vi "clone.vi"(0 "reference":refnum<class "PackageNode.lvclass">, 5 "error in (no error)":errorcluster) -> (14 "reference out":refnum<class "PackageNode.lvclass">, 15 "clonedPackageNode":refnum<class "AbstractNode.lvclass">, 19 "error out":errorcluster)   [LabVIEW 2020, in "PackageNode.lvclass"]
doc: "public Object clone()"
uses:
  <resource>/Framework/Providers/Open_GDS/UML/PackageNode_class/PackageNode.lvclass
  C:/Program Files (x86)/National Instruments/LabVIEW 2020/resource/Framework/Providers/Open_GDS/UML/RectangularNode_class/RectangularNode.lvclass
  C:/Program Files (x86)/National Instruments/LabVIEW 2020/resource/Framework/Providers/Open_GDS/UML/AbstractNode_class/AbstractNode.lvclass
  <resource>/Framework/Providers/Open_GDS/UML/AbstractNode_class/AbstractNode.lvclass
  <resource>/Framework/Providers/Open_GDS/UML/MultiLineString_class/MultiLineString.lvclass
  <resource>/Framework/Providers/Open_GDS/UML/RectangularNode_class/RectangularNode.lvclass
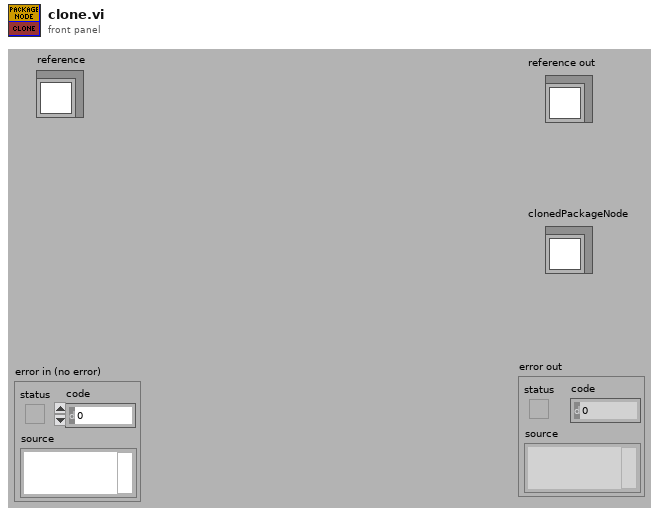
[diagram p1: front panel]
types:
  T1 = typedef "PackageNode.lvclass/ObjectAttributes.ctl" = cluster{"name":string, "contents":refnum<class "MultiLineString.lvclass">, "DEFAULT_TOP_WIDTH":i32, "DEFAULT_TOP_HEIGHT":i32, "DEFAULT_WIDTH":i32, "DEFAULT_HEIGHT":i32, "NAME_GAP":i32, "XGAP":i32, "YGAP":i32, "Collapsed":bool, "Note color":u32, "Justification":u16}
  T2 = typedef "RectangularNode.lvclass/ObjectAttributes.ctl" = cluster{"bounds":T3}
  T3 = typedef "Rectangle Rectangle2D.ctl" = cluster{"x":dbl, "y":dbl, "width":dbl, "height":dbl}
  T4 = typedef "AbstractNode.lvclass/ObjectAttributes.ctl" = cluster{"parent":refnum<class "AbstractNode.lvclass">, "children":refnum<class "AbstractNode.lvclass">[], "Hidden":bool}
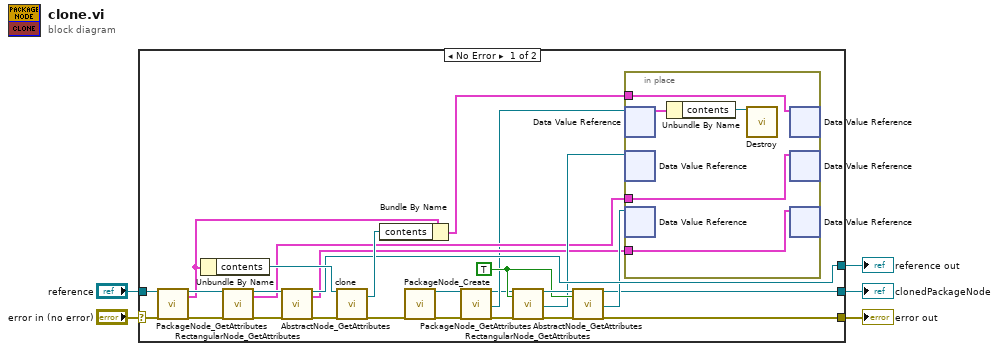
[diagram p0: block diagram]
diagram:
  n1 = case shown="No Error" "error in (no error)" {
    selector: "error in (no error)" -> [w16 w38]
    tunnel: "reference" -> [w15 w39]
    tunnel: [w20 w38] -> w1
    tunnel: [w28 w39] -> w2
    tunnel: [w19 _] -> w3
    frame No Error {
      w23 = TRUE ("OnlyGetDvrReference(False)")
      n2 = call <resource>:"PackageNode_GetAttributes.vi"("reference in"=w15, "error in (no error)"=w16) -> ("reference out"=w13:refnum<class "PackageNode.lvclass">, "Data"=w12:T1, "error out"=w14:errorcluster)  [unwired: 1 in, 14 out]
      n3 = Unbundle By Name(w12) -> ("contents"=w32:refnum<class "MultiLineString.lvclass">)
      n4 = call <resource>:"RectangularNode_GetAttributes.vi"("reference in"=w13, "error in (no error)"=w14) -> ("reference out"=w29:refnum<class "PackageNode.lvclass">, "Data"=w18:T2, "error out"=w27:errorcluster)  [unwired: 14 in, 1 out]
      n5 = call <resource>:"AbstractNode_GetAttributes.vi"("reference in"=w29, "error in (no error)"=w27) -> ("reference out"=w28:refnum<class "PackageNode.lvclass">, "Data"=w17:T4, "error out"=w26:errorcluster)  [unwired: 14 in, 1 out]
      n6 = call-dynamic "clone.vi"("reference"=w32, "error in (no error)"=w26) -> ("clonedMultiLineString"=w31:refnum<class "MultiLineString.lvclass">, "error out"=w11:errorcluster)  [unwired: 15 in, 1 out]
      n7 = Bundle By Name(cluster=w12, "contents"=w31) -> (w30:T1)
      n8 = call <resource>:"PackageNode_Create.vi"("error in (no error)"=w11) -> ("reference out"=w10:refnum<class "PackageNode.lvclass">, "error out"=w9:errorcluster)  [unwired: 17 in]
      n9 = call <resource>:"PackageNode_GetAttributes.vi"("reference in"=w10, "error in (no error)"=w9) -> ("reference out"=w6:refnum<class "PackageNode.lvclass">, "DataRef"=w7:refnum<data-value>, "error out"=w8:errorcluster)  [unwired: 1 in, 14 out]
      n10 = call <resource>:"RectangularNode_GetAttributes.vi"("reference in"=w6, "OnlyGetDvrReference(False)"=w23, "error in (no error)"=w8) -> ("reference out"=w24:refnum<class "PackageNode.lvclass">, "DataRef"=w22:refnum<data-value>, "error out"=w25:errorcluster)  [unwired: 13 in, 1 out]
      n11 = call <resource>:"AbstractNode_GetAttributes.vi"("reference in"=w24, "OnlyGetDvrReference(False)"=w23, "error in (no error)"=w25) -> ("reference out"=w19:refnum<class "PackageNode.lvclass">, "DataRef"=w21:refnum<data-value>, "error out"=w20:errorcluster)  [unwired: 13 in, 1 out]
      n12 = in-place {
        in-place-border: w30 -> [w37]
        in-place-border: w18 -> [w36]
        in-place-border: w17 -> [w35]
        n13 = in-place-dvr #1(w7) -> (w33:T1)  [unwired: 1 out]
        n14 = in-place-dvr #2(w22) -> ()  [unwired: 2 out]
        n15 = in-place-dvr #3(w21) -> ()  [unwired: 2 out]
        n16 = Unbundle By Name(w33) -> ("contents"=w34:refnum<class "MultiLineString.lvclass">)
        n17 = call-dynamic "Destroy.vi"("reference"=w34) -> ()  [unwired: 17 in, 2 out]
        n18 = in-place-dvr #1(w37) -> ()  [unwired: 2 out]
        n19 = in-place-dvr #2(w36) -> ()  [unwired: 2 out]
        n20 = in-place-dvr #3(w35) -> ()  [unwired: 2 out]
      }
    }
    frame Error {
    }
  }
  "reference out" <- w2
  "error out" <- w1
  "clonedPackageNode" <- w3
